vi "Average_IB_curves.vi"(0 "I in":dbl[](array[numeric]), 2 "Counter":i8, 5 "Averaged I(B) In":dbl[][](array[numeric]), 9 "B in":dbl[](array[numeric]), 12 "Up/Down":bool, 14 "B array":dbl[](array[numeric])) -> (4 "Averaged I(B) out":dbl[][](array[numeric]))   [LabVIEW 2015]
uses:
  <vilib>/Analysis/baseanly.llb/Mean (DBL).vi
  <vilib>/Analysis/NI_AALBase.lvlib
panel:
  out "Down":cluster{"B array":dbl[], dbl[]}(graph)
  out "XY Graph 2":cluster{"B in":dbl[], "I in":dbl[]}(graph)
  out "Up":cluster{"B array":dbl[], dbl[]}(graph)
  out "subarray 2":dbl[](array[numeric])
  out "subarray":dbl[](array[numeric])
  out "Sorted array":dbl[][](array[numeric]) format="%.5f"
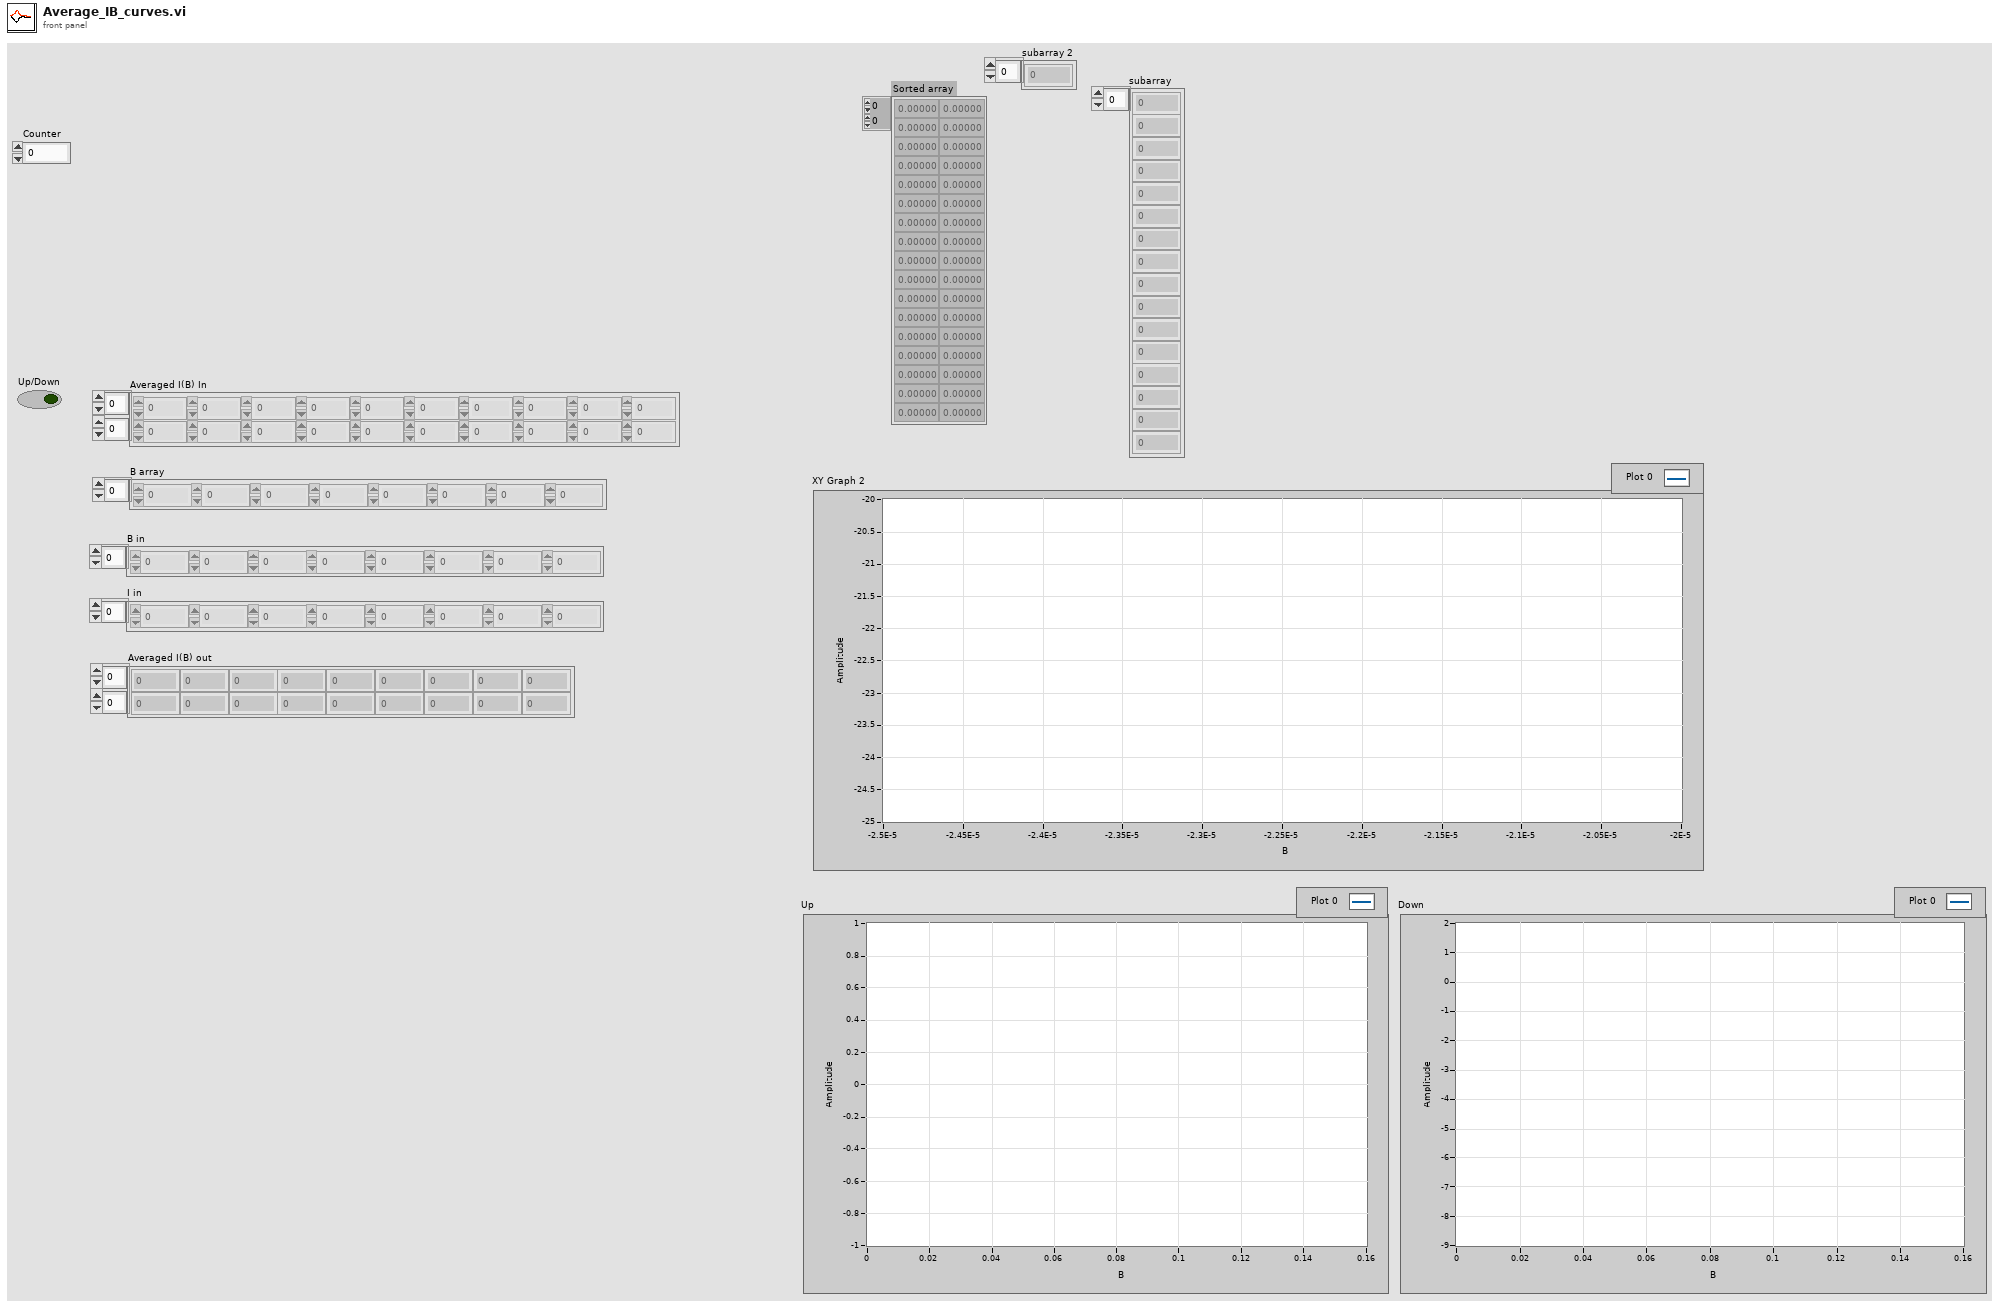
[diagram p1: front panel]
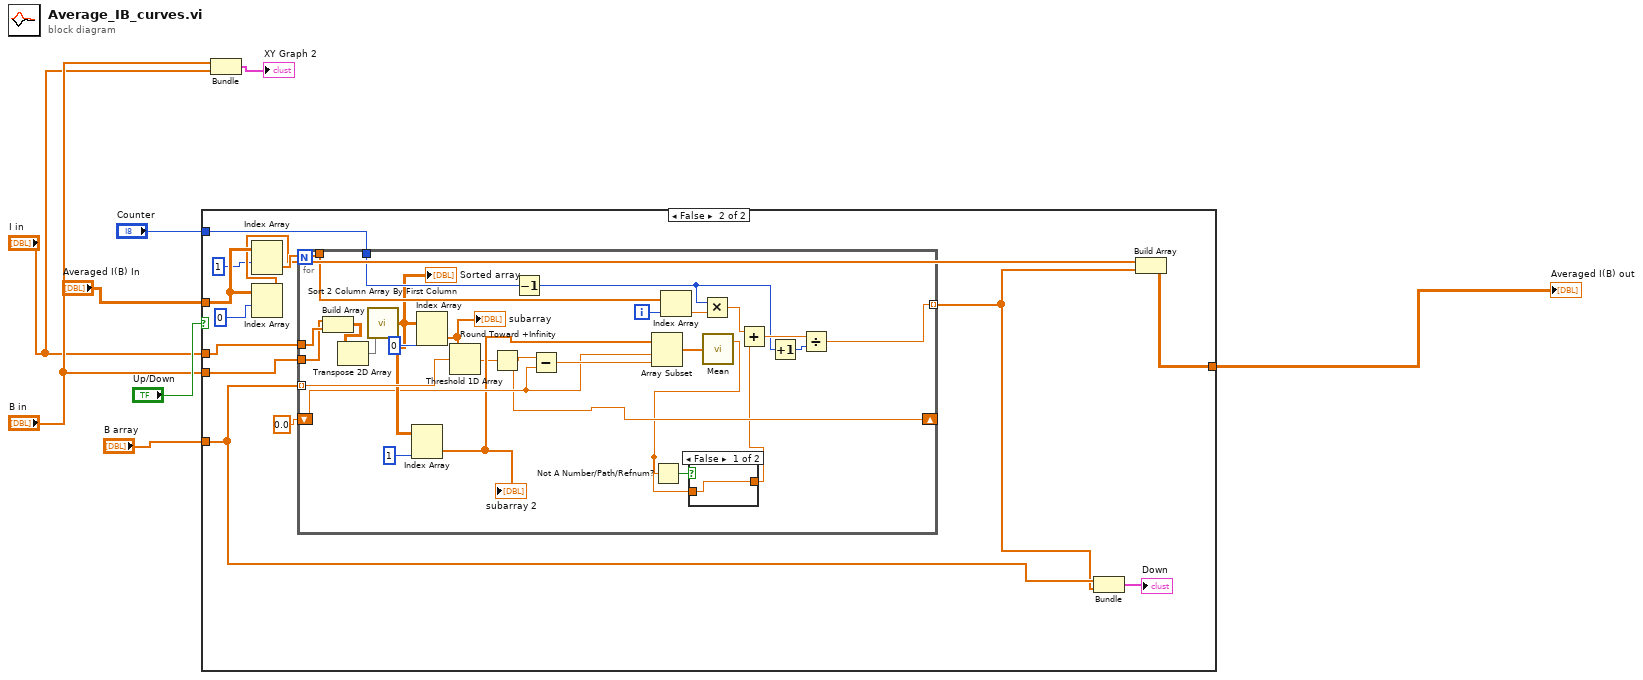
[diagram p0: block diagram]
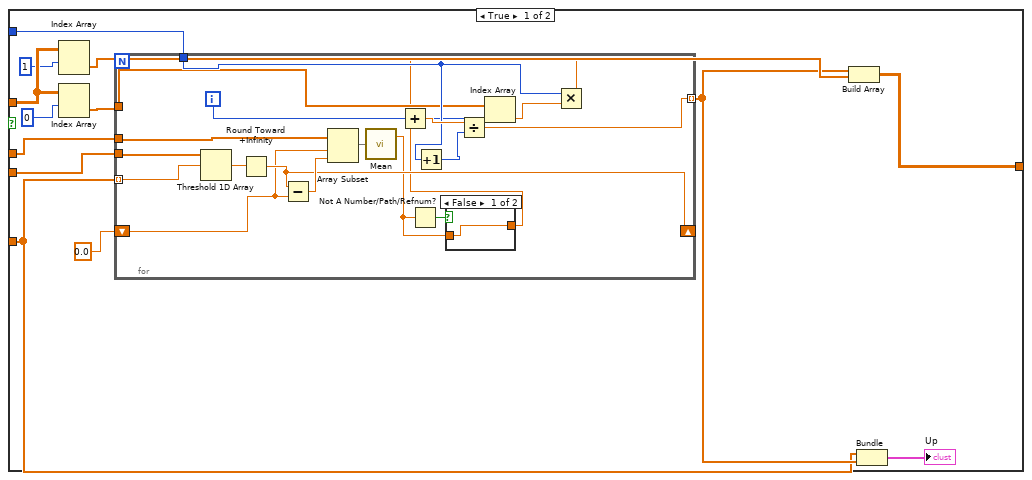
[diagram p2: hidden frame]
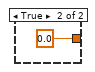
[diagram p3: hidden frame]
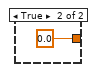
[diagram p4: hidden frame]
diagram:
  n1 = case shown="False" "Up/Down" {
    tunnel: "Averaged I(B) In" -> [w16 w51]
    tunnel: "I in" -> [w18 w53]
    tunnel: "B in" -> [w20 w55]
    tunnel: "Counter" -> [w17 w52]
    tunnel: "B array" -> [w10 w45]
    tunnel: [w15 w50] -> w8
    frame True {
      n2 = Index Array(array=w16, index (row)=1 ("disabled index (col)")) -> (element=w12:dbl[])  [unwired: 1 in]
      n3 = Index Array(array=w16, index (row)=0 ("disabled index (col)")) -> (element=w21:dbl[])  [unwired: 1 in]
      n4 = for {
        tunnel: w21 -> [w33]
        tunnel: w10 -> [w23] mode=indexing
        tunnel: w20 -> [w40]
        shift-right: [w28] -> _
        shift-left: 0.0 -> [w27]
        tunnel: w18 -> [w39]
        tunnel: w17 -> [w35]
        tunnel: [w34] -> w11 mode=indexing
        i -> [w32]
        n5 = Threshold 1D Array(2:w23, 3:w40) -> (0:w29:dbl)  [unwired: 1 in]
        n6 = Round Toward +Infinity(x=w29) -> (ceil(x): smallest int >= x=w28:dbl)
        n7 = Subtract(x=w28, y=w27) -> (x-y=w38:dbl)
        n8 = Array Subset(array=w39, index=w27, length=w38) -> (w30:dbl[])
        n9 = call-poly <vilib>:"Mean.vi"("X"=w30) -> ("mean"=w25:dbl)  [unwired: 1 out]
        n10 = Not A Number/Path/Refnum?(number/path/refnum=w25) -> (NaN/Path/Refnum?=w26:bool)
        n11 = Increment(x=w35) -> (x+1=w36:i8)
        n12 = case shown="False" w26 {
          tunnel: [w41 0.0] -> w24
          tunnel: w25 -> [w41 _]
          frame False {
          }
          frame True {
          }
        }
        n13 = Index Array(array=w33, index=w32) -> (element=w31:dbl)
        n14 = Multiply(x=w35, y=w31) -> (x*y=w22:dbl)
        n15 = Add(x=w22, y=w24) -> (x+y=w37:dbl)
        n16 = Divide(x=w37, y=w36) -> (x/y=w34:dbl)
      }
      n17 = Build Array(w11, w12) -> (w15:dbl[][])
      n18 = Bundle("B array"=w10, w11) -> (→"Up":cluster{"B array":dbl[], dbl[]})  [unwired: 1 in]
    }
    frame False {
      n19 = Index Array(array=w51, index (row)=1 ("disabled index (col)")) -> (element=w49:dbl[])  [unwired: 1 in]
      n20 = Index Array(array=w51, index (row)=0 ("disabled index (col)")) -> (element=w48:dbl[])  [unwired: 1 in]
      n21 = for {
        tunnel: w49 -> [w76]
        tunnel: w45 -> [w82] mode=indexing
        tunnel: w55 -> [w71]
        shift-right: [w61] -> _
        shift-left: 0.0 -> [w64]
        tunnel: w53 -> [w72]
        tunnel: w52 -> [w77]
        tunnel: [w56] -> w44 mode=indexing
        i -> [w75]
        n22 = Build Array(w71, w72) -> (w66:dbl[][])
        n23 = Transpose 2D Array(2D array=w66) -> (transposed array=w65:dbl[][])
        n24 = call "Sort 2 Column Array By First Column.vi"("2D array to sort"=w65) -> ("Sorted array"=w68:dbl[][])
        "Sorted array" <- w68
        n25 = Index Array(array=w68, index (col)=1 ("disabled index (col)")) -> (element=w63:dbl[])  [unwired: 1 in]
        "subarray 2" <- w63
        n26 = Index Array(array=w68, index (col)=0 ("disabled index (col)")) -> (element=w70:dbl[])  [unwired: 1 in]
        "subarray" <- w70
        n27 = Threshold 1D Array(2:w82, 3:w70) -> (0:w62:dbl)  [unwired: 1 in]
        n28 = Round Toward +Infinity(x=w62) -> (ceil(x): smallest int >= x=w61:dbl)
        n29 = Decrement(x=w77) -> (x-1=w57:i8)
        n30 = Subtract(x=w61, y=w64) -> (x-y=w81:dbl)
        n31 = Array Subset(array=w63, index=w64, length=w81) -> (w73:dbl[])
        n32 = Index Array(array=w76, index=w75) -> (element=w74:dbl)
        n33 = Multiply(x=w57, y=w74) -> (x*y=w80:dbl)
        n34 = call-poly <vilib>:"Mean.vi"("X"=w73) -> ("mean"=w59:dbl)  [unwired: 1 out]
        n35 = Not A Number/Path/Refnum?(number/path/refnum=w59) -> (NaN/Path/Refnum?=w60:bool)
        n36 = case shown="False" w60 {
          tunnel: [w83 0.0] -> w58
          tunnel: w59 -> [w83 _]
          frame False {
          }
          frame True {
          }
        }
        n37 = Add(x=w80, y=w58) -> (x+y=w79:dbl)
        n38 = Increment(x=w57) -> (x+1=w78:i8)
        n39 = Divide(x=w79, y=w78) -> (x/y=w56:dbl)
      }
      n40 = Bundle("B array"=w45, w44) -> (→"Down":cluster{"B array":dbl[], dbl[]})  [unwired: 1 in]
      n41 = Build Array(w48, w44) -> (w50:dbl[][])
    }
  }
  "Averaged I(B) out" <- w8
  n42 = Bundle("B in"="B in", "I in"="I in") -> (→"XY Graph 2":cluster{"B in":dbl[], "I in":dbl[]})  [unwired: 1 in]
